vi "RenameValiseFiles.vi"(4 "Error In":errorcluster caption="Entrée d'erreur", 6 "NumEssai":u32, 7 "NomProjet":string) -> (0 "sortie d'erreur":errorcluster, 2 "NewValiseFile":path, 3 "NomProjetOut":string)   [LabVIEW 2015]
uses:
  DefDeType/WhichPath.ctl
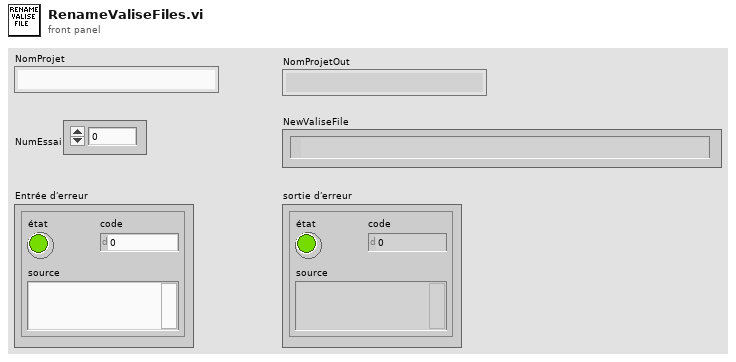
[diagram p1: front panel]
types:
  T1 = typedef "WhichPath.ctl" = enum16{"DossierProjet", "Config", "Meas", "MeasSuitCase", "MeasOnBoard", "MeasQualisys", "MeasTDMS", "MeasHexapode", "MeasNortek", "Fig", "Res"}
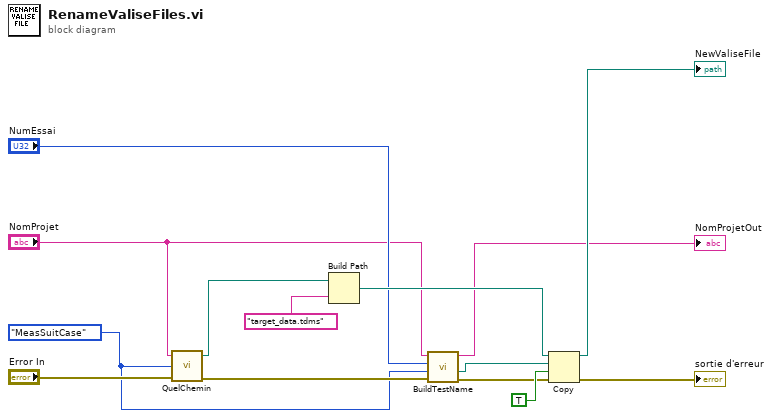
[diagram p0: block diagram]
diagram:
  w2 = WhichPath."MeasSuitCase" ("WhichPath?")
  n1 = call "QuelChemin.vi"("Entrée d'erreur"="Error In", "WhichPath?"=w2, "NomProjet"="NomProjet") -> ("Sortie d'erreur"=w8:errorcluster, "SurDisqueLocal"=w3:path)  [unwired: 1 out]
  n2 = Build Path(base path=w3, name or relative path="target_data.tdms" ("remote path")) -> (appended path=w13:path)
  n3 = call "BuildTestName.vi"("entrée d'erreur"=w8, "WhichPath?"=w2, "NextTestNum"="NumEssai", "NomProjet"="NomProjet") -> ("sortie d'erreur"=w9:errorcluster, "cheminProchainFichier"=w5:path, "NomProjetOut"=→"NomProjetOut":string)  [unwired: 1 in, 1 out]
  n4 = Copy(8:w9, 9:TRUE ("écraser (F)"), 10:w5, 11:w13) -> (0:→"sortie d'erreur":errorcluster, 3:→"NewValiseFile":path)  [unwired: 1 in, 1 out]
